vi "New.vi"(5 "FIFO Options":T1, 7 "id (0)":i32, 8 "error in (no error)":errorcluster, 9 "fifo depths (10)":u32=10, 10 "error size (512 B)":T2=enum."512-byte", 11 "Plugin Interface type":refnum<class "Plugin Interface.lvclass">) -> (0 "error out":errorcluster, 3 "Plugin Interface":refnum<class "Plugin Interface.lvclass">)   [LabVIEW 2017, in "DSF Core.lvlib" / "Plugin Interface.lvclass"]
uses:
  Plugin Interface.lvclass
  C:/Git/DSF/Data Sharing Framework/Source/Core/Engine/Classes/Interfaces/Interface/Interface.lvclass
  Interface/Error Queue Sizes.ctl
  Typedefs/FIFO Flags.ctl
  Interface/Interface.lvclass
  DSF Core.lvlib
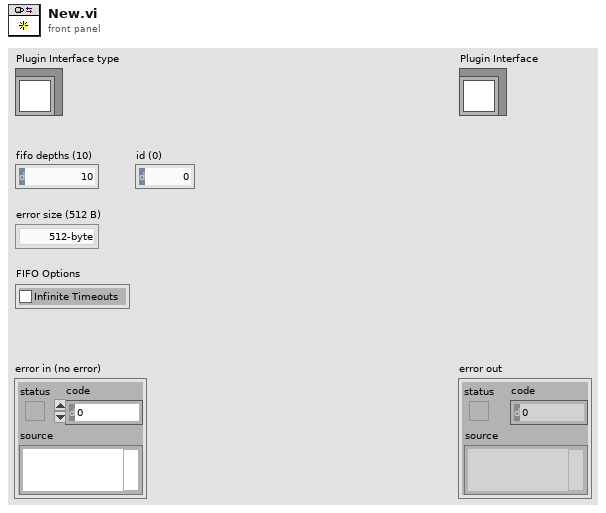
[diagram p1: front panel]
types:
  T1 = typedef "DSF Core.lvlib/FIFO Flags.ctl" = cluster{"Infinite Timeouts":bool}
  T2 = typedef "DSF Core.lvlib/Interface.lvclass/Error Queue Sizes.ctl" = enum16{"256-byte", "512-byte", "1024-byte"}
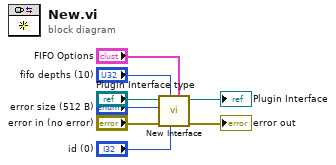
[diagram p0: block diagram]
diagram:
  n1 = call "New Interface.vi"("FIFO Options"="FIFO Options", "id (0)"="id (0)", "fifo/queue depths (10)"="fifo depths (10)", "error in (no error)"="error in (no error)", "error size (512 B)"="error size (512 B)", "Interface type"="Plugin Interface type") -> ("error out"=→"error out":errorcluster, "Interface"=→"Plugin Interface":refnum<class "Plugin Interface.lvclass">)  [unwired: 4 in]
